vi "Get Pressure Servo Valve Settings.vi"(11 "ILC Actuator Cylinder in":refnum<class "ILC Actuator Cylinder.lvclass">) -> (2 "Pressure Servo Settings":T1={"Center Point"=2.5, "Area"=0.004536, "PA to PSI"=0.000145038, "Off Value"=0.004536} {"Off Value" format="%.3f"; "PA to PSI" format="%.9f"; "Area" format="%.9f"; "Center Point" format="%.3f"}, 3 "ILC Actuator Cylinder out":refnum<class "ILC Actuator Cylinder.lvclass">)   [LabVIEW 2015, in "ILC Actuator Cylinder.lvclass"]
uses:
  ILC Actuator Cylinder.lvclass
  Typedefs/Pressure Servo Valve Settings.ctl
  ILC Actuator Cylinder.lvclass/ILC Actuator Cylinder.ctl
  Typedefs/FAMT Typedefs.lvlib
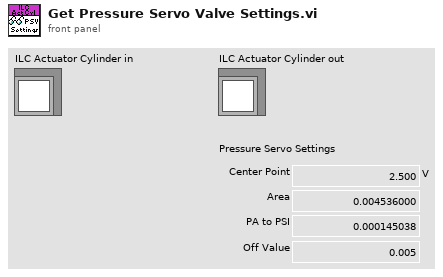
[diagram p1: front panel]
types:
  T1 = typedef "FAMT Typedefs.lvlib/Pressure Servo Valve Settings.ctl" = cluster{"Center Point":dbl[unit], "Area":dbl, "PA to PSI":dbl, "Off Value":dbl}
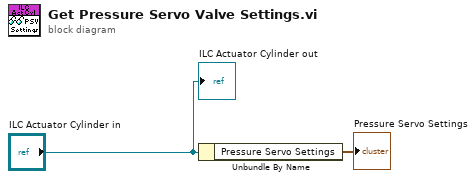
[diagram p0: block diagram]
diagram:
  n1 = Unbundle By Name("ILC Actuator Cylinder in") -> ("Pressure Servo Settings"=→"Pressure Servo Settings":T1)
  "ILC Actuator Cylinder out" <- "ILC Actuator Cylinder in"
